vi "Configure Level.vi"(0 "VISA resource name":refnum<visa-resource-name>, 1 "Reference Level Offset (0 dB)":dbl, 2 "Enable Input Port Power Gain (T: Enable)":bool=TRUE, 5 "Amplitude Units (0: dBm)":i32(ring) items=["dBm", "dBmV", "dBmVEMF", "dBuV", "dBuVEMF", "V", "W", "VEMF"], 7 "Reference Level (0 dBm)":i32, 9 "Manual Attenuation (20 dB)":dbl=20.0, 11 "error in (no error)":errorcluster, 12 "Auto Attenuation (T: Enable)":bool=TRUE, 13 "Enable High Sensitivity (T: Enable)":bool=TRUE) -> (4 "VISA resource name out":refnum<visa-resource-name>, 15 "error out":errorcluster)   [LabVIEW 2022 SP3, in "Agilent N934X Series.lvlib"]
doc: "Configures the vertical settings of the spectrum analyzer."
uses:
  <instrlib>/Agilent N934X Series/Agilent N934X Series.lvlib
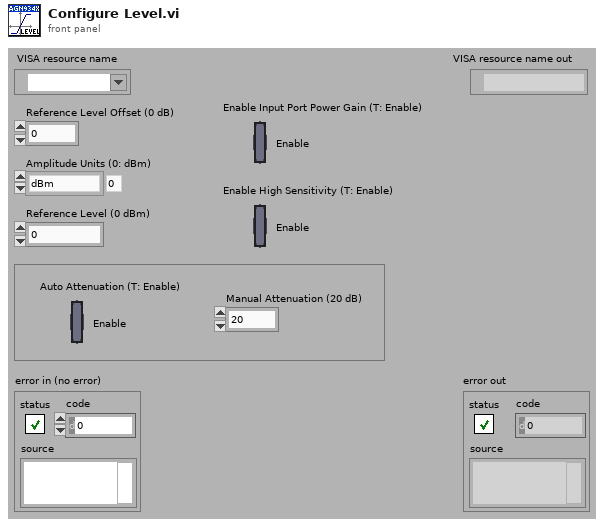
[diagram p1: front panel]
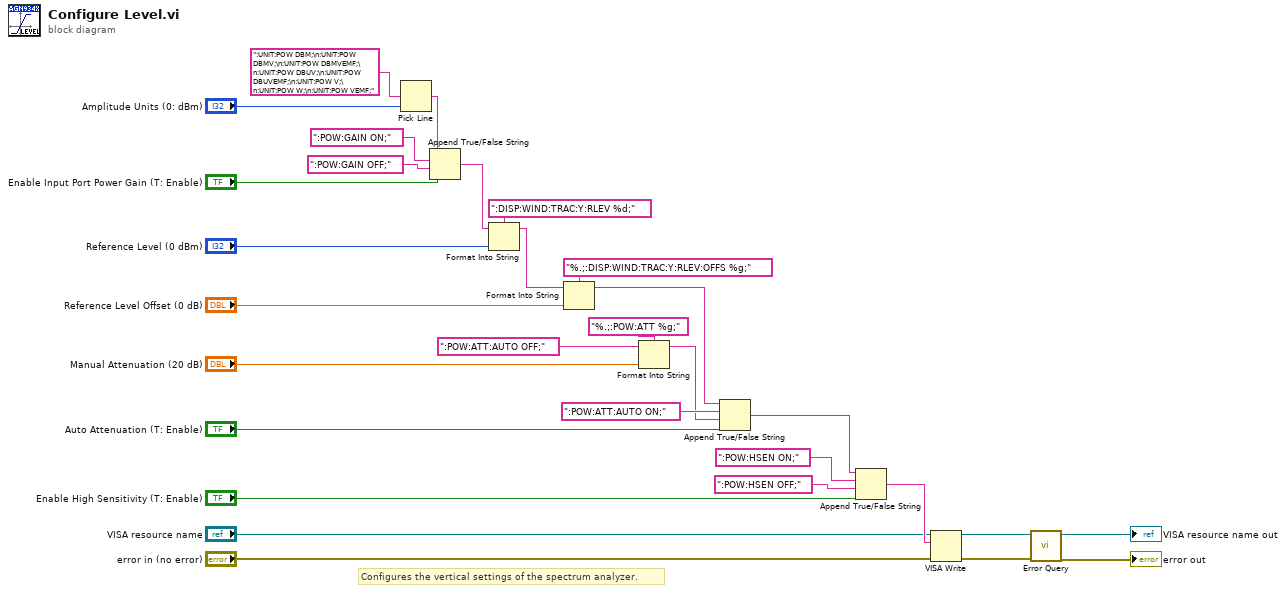
[diagram p0: block diagram]
diagram:
  # "Configures the vertical settings of the spectrum analyzer."
  n1 = Pick Line(multi-line string=":UNIT:POW DBM;\n:UNIT:POW DBMV;\n:UNIT:POW DBMVEMF;\n:UNIT:POW DBUV;\n:UNIT:POW DBUVEMF;\n:UNIT:POW V;\n:UNIT:POW W;\n:UNIT:POW VEMF;", line index="Amplitude Units (0: dBm)") -> (output string=w3:string)  [unwired: 1 in]
  n2 = Append True/False String(1:"Enable Input Port Power Gain (T: Enable)", 2:":POW:GAIN OFF;", 3:":POW:GAIN ON;", 4:w3) -> (0:w2:string)
  n3 = Format Into String(format string=":DISP:WIND:TRAC:Y:RLEV %d;", initial string=w2, "Reference Level (0 dBm)") -> (resulting string=w28:string)  [unwired: 1 in, 1 out]
  n4 = Format Into String(format string="%.;:DISP:WIND:TRAC:Y:RLEV:OFFS %g;", initial string=w28, "Reference Level Offset (0 dB)") -> (resulting string=w6:string)  [unwired: 1 in, 1 out]
  n5 = Format Into String(format string="%.;:POW:ATT %g;", initial string=":POW:ATT:AUTO OFF;", "Manual Attenuation (20 dB)") -> (resulting string=w7:string)  [unwired: 1 in, 1 out]
  n6 = Append True/False String(1:"Auto Attenuation (T: Enable)", 2:w7, 3:":POW:ATT:AUTO ON;", 4:w6) -> (0:w1:string)
  n7 = Append True/False String(1:"Enable High Sensitivity (T: Enable)", 2:":POW:HSEN OFF;", 3:":POW:HSEN ON;", 4:w1) -> (0:w16:string)
  n8 = VISA Write(VISA resource name="VISA resource name", write buffer=w16, error in (no error)="error in (no error)") -> (VISA resource name out=w13:refnum<visa-resource-name>, error out=w12:errorcluster)  [unwired: 1 out]
  n9 = call <instrlib>:"Error Query.vi"("error in (no error)"=w12, "VISA resource name"=w13) -> ("error out"=→"error out":errorcluster, "VISA resource name out"=→"VISA resource name out":refnum<visa-resource-name>)  [unwired: 6 in, 2 out]
